vi "Destroy Buffer.vi"(8 "error in (no error)":errorcluster, 11 "Circular Buffer 1D U16 DVR Queue in":refnum<class "Circular Buffer 1D U16 DVR Queue.lvclass">) -> (0 "error out":errorcluster, 3 "Circular Buffer 1D U16 DVR Queue out":refnum<class "Circular Buffer 1D U16 DVR Queue.lvclass">)   [LabVIEW 2019, in "Circular Buffer 1D U16 DVR Queue.lvclass"]
uses:
  Circular Buffer 1D U16 DVR Queue.lvclass
  Circular Buffer 1D U16 DVR Queue.lvclass/Circular Buffer 1D U16 DVR Queue.ctl
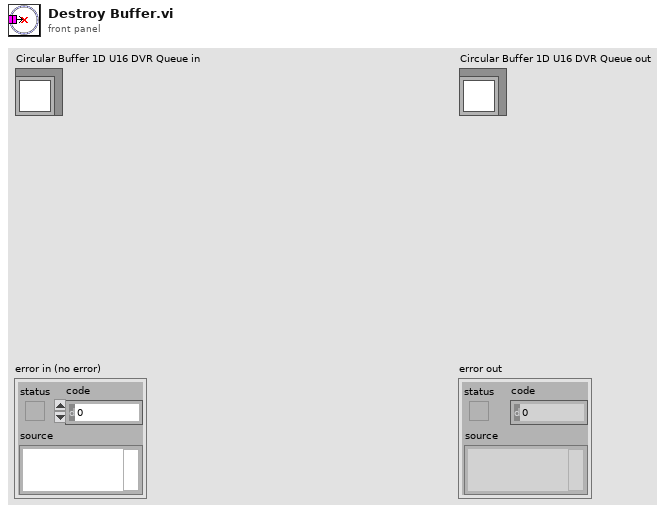
[diagram p1: front panel]
types:
  T1 = typedef "1D U16 DVR Queue.ctl" = refnum<queue>
  T2 = typedef "1D U16 DVR.ctl" = refnum<data-value>
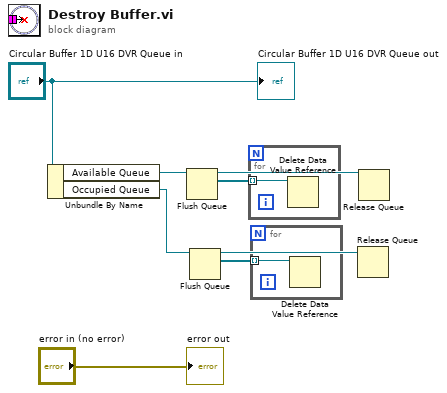
[diagram p0: block diagram]
diagram:
  n1 = Unbundle By Name("Circular Buffer 1D U16 DVR Queue in") -> ("Available Queue"=w6:T1, "Occupied Queue"=w5:T1)
  n2 = Flush Queue(queue=w6) -> (queue out=w3:T1, remaining elements=w4:T2[])  [unwired: 1 in, 1 out]
  n3 = Flush Queue(queue=w5) -> (queue out=w1:T1, remaining elements=w2:T2[])  [unwired: 1 in, 1 out]
  n4 = for {
    tunnel: w4 -> [w9] mode=indexing
    n5 = Delete Data Value Reference(data value reference=w9) -> ()  [unwired: 1 in, 2 out]
  }
  n6 = for {
    tunnel: w2 -> [w10] mode=indexing
    n7 = Delete Data Value Reference(data value reference=w10) -> ()  [unwired: 1 in, 2 out]
  }
  n8 = Release Queue(queue=w1) -> ()  [unwired: 2 in, 3 out]
  n9 = Release Queue(queue=w3) -> ()  [unwired: 2 in, 3 out]
  "error out" <- "error in (no error)"
  "Circular Buffer 1D U16 DVR Queue out" <- "Circular Buffer 1D U16 DVR Queue in"
